vi "Process Sink Error.vi"(10 "Error To Process":errorcluster, 11 "Log Sink in":refnum<class "Log Sink.lvclass">) -> (0 "error out":errorcluster, 3 "Log Sink out":refnum<class "Log Sink.lvclass">, 4 "Stop Sink?":bool)   [LabVIEW 2020, in "MVA Framework.lvlib" / "Composed Log.lvlib" / "Log Sink.lvclass"]
uses:
  Log Sink.lvclass
  Log Sink.lvclass/Log Sink.ctl
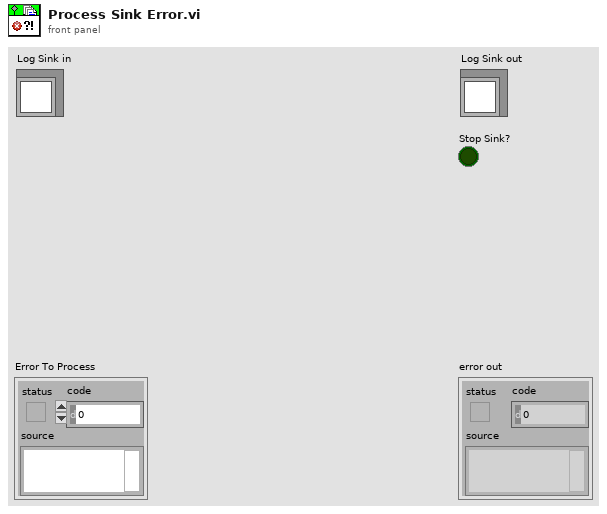
[diagram p1: front panel]
types:
  T1 = typedef "MVA Framework.lvlib/Composed Log.lvlib/Log Sink.lvclass/Sink Error Actions ENUM.ctl" = enum16{"Ignore Error and Continue", "Ignore Error and Close Sink", "Report Error and Close Sink"}
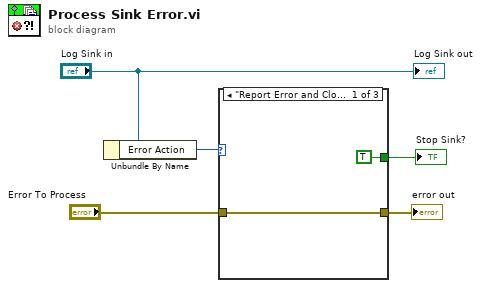
[diagram p0: block diagram]
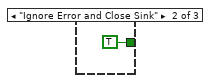
[diagram p2: hidden frame]
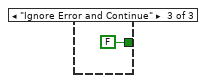
[diagram p3: hidden frame]
diagram:
  n1 = Unbundle By Name("Log Sink in") -> ("Error Action"=w1:T1)
  n2 = case shown="\"Report Error and Close Sink\"" w1 {
    tunnel: "Error To Process" -> [w7 _ _]
    tunnel: [TRUE TRUE FALSE] -> w4
    tunnel: [w7 _ _] -> w3
    frame "Report Error and Close Sink" {
    }
    frame "Ignore Error and Close Sink" {
    }
    frame "Ignore Error and Continue" {
    }
  }
  "error out" <- w3
  "Stop Sink?" <- w4
  "Log Sink out" <- "Log Sink in"
